vi "ziExample-PWA_SignalInput.vi"() -> ()   [LabVIEW 2009]
doc: "Control a Zurich instrument device via the LabOne Labview API. \nRequirements: Zurich Instruments UHFLI \nThis example retrives Periodic Waveform Analyzer (PWA) data from an UHFLI instrument.\n\n© Zurich Instruments AG, www.zhinst.com\\"
uses:
  <instrlib>/Zurich Instruments LabOne/Public/Data/ziTypePWAWave.ctl
  <instrlib>/Zurich Instruments LabOne/Public/Configure/ziGetValueString.vi
  <instrlib>/Zurich Instruments LabOne/Public/Configure/ziSetValueDoubleArray.vi
  <vilib>/Analysis/2dsp.llb/Real FFT.vi
  <instrlib>/Zurich Instruments LabOne/Public/Data/ziGetEventPWAWave.vi
  <instrlib>/Zurich Instruments LabOne/Zurich Instruments LabOne.lvlib
  <vilib>/Analysis/NI_AALPro.lvlib
  <vilib>/Analysis/NI_AALBase.lvlib
panel:
  out "Error Out":errorcluster
  out "Selected Device":string
  in  "Address":string="DEV"
  in  "Bins":i32=512
  in  "stop":bool
  out "PWAWave":T1={"Timestamp (ticks)"=2149, "SampleCount"=0, "InputSelect"=0, "OscSelect"=0, "Harmonic"=0, "BinCount"=0, "Frequency (Hz)"=0.0, "PWAType"=0, "Mode"=0, "Overflow"=0, "Commensurable"=0, "BinPhase"=[], "X"=[], "Y"=[], "countBin"=[]} {"Frequency (Hz)" format="%#_6p"}
  out "FFT / Harmonics":dbl[](graph)
  out "Waveform":cluster{dbl[], dbl[]}(graph)
  out "Counts per Bin":cluster{dbl[], u32[]}(graph)
  # "ziExample-PWA.vi\nRequirements: UHFLI + BOX\nOptional: MF\nsee block diagram for VI description"
  # "Tested Devices:\n- UHFLI"
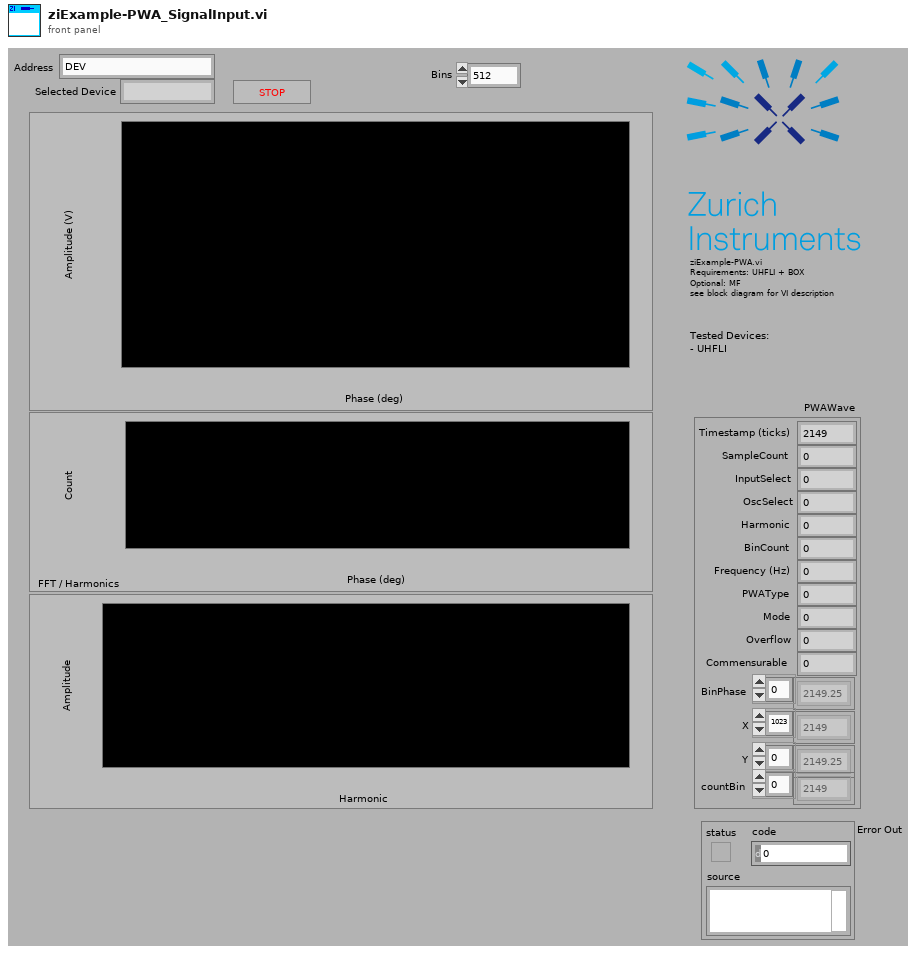
[diagram p1: front panel]
types:
  T1 = typedef "Zurich Instruments LabOne.lvlib/ziTypePWAWave.ctl" = cluster{"Timestamp (ticks)":u64, "SampleCount":u64, "InputSelect":i32, "OscSelect":i32, "Harmonic":i32, "BinCount":i32, "Frequency (Hz)":dbl, "PWAType":u8, "Mode":u8, "Overflow":u8, "Commensurable":u8, "BinPhase":dbl[], "X":dbl[], "Y":dbl[], "countBin":u32[]}
  T2 = typedef "Zurich Instruments LabOne.lvlib/ziTypeHandle.ctl" = cluster{"handleValid":bool, "Conn":u64, "Path Prefix":string, "Handle":u64, "Connected":bool, "Clockbase(s)":dbl}
  T3 = typedef "Zurich Instruments LabOne.lvlib/ziTypePollType.ctl" = enum16{"NONE", "DOUBLE_DATA", "INTEGER_DATA", "DEMOD_SAMPLE", "SCOPE_WAVE_HF2", "AUXIN_SAMPLE", "DIO_SAMPLE", "BYTE_ARRAY", "PWA_WAVE", "9", "10", "11", "12", "13", "14", "15", "TREE_CHANGE_DEPRI", "17", "ERROR", "19", "20", "21", "22", "23", "24", "25", "26", "27", "28", "29", "30", "31", "DOUBLE_DATA_TS", "INTEGER_DATA_TS", "34", "SCOPE_WAVE", "SCOPE_WAVE_EX", "37", "BYTE_ARRAY_TS", "39", "40", "41", "42", "43", "44", "45", "CNT_DATA", "47", "TREE_CHANGE", "49", "50", "51", "52", "53", "54", "55", "56", "57", "58", "59", "60", "61", "62", "63", "SWEEPER_DATA", "SPECTRUM_DATA", "ADVISOR_DATA", "VECTOR_DATA", "IMP_DATA"}
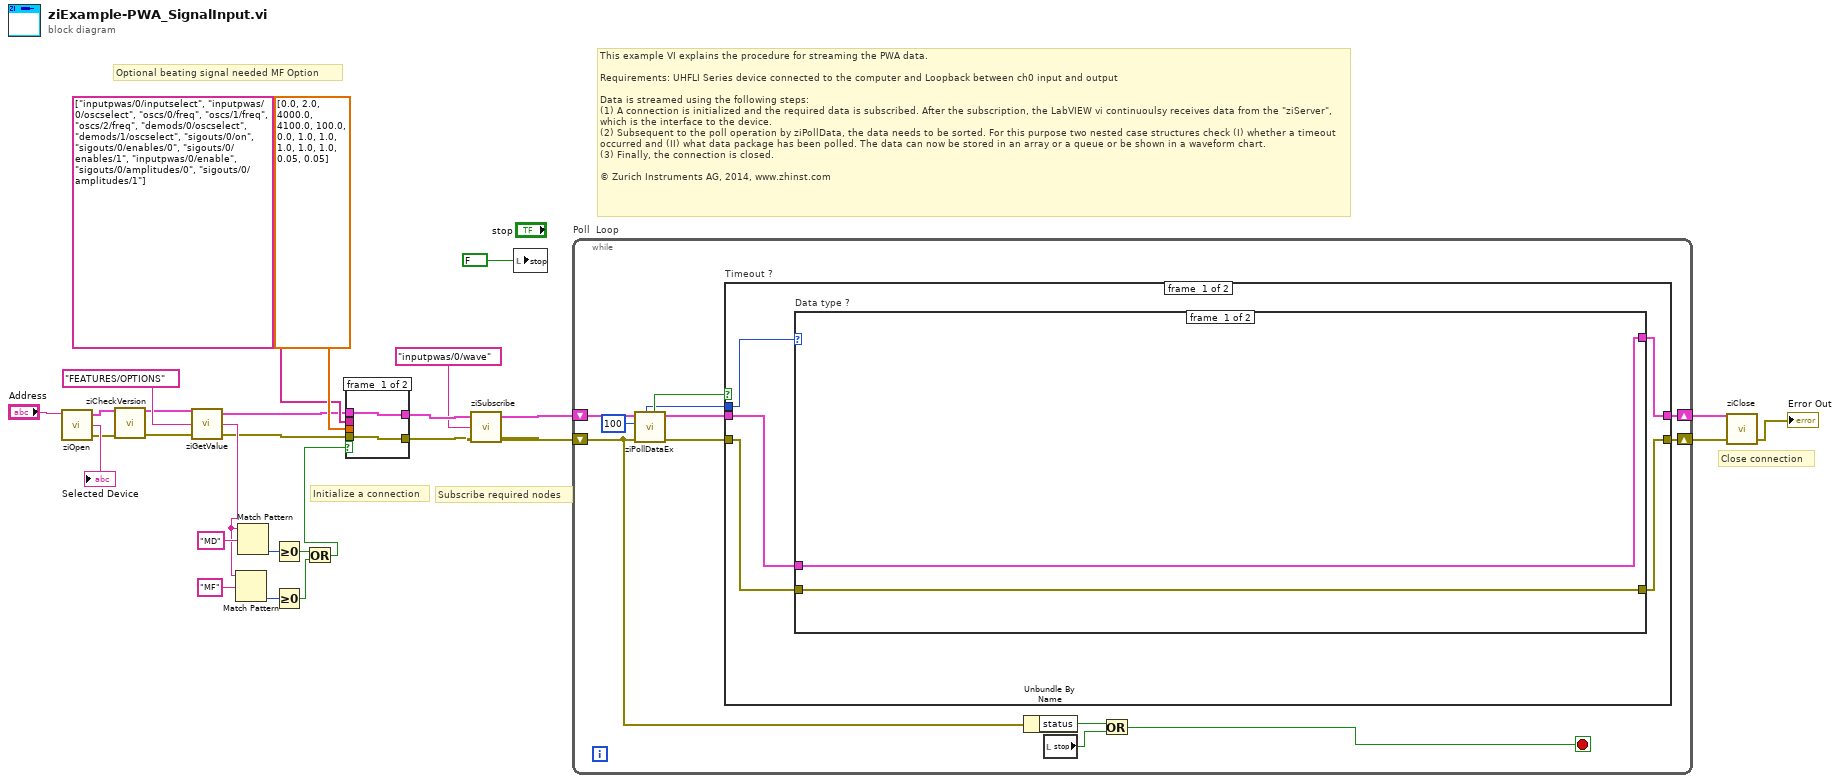
[diagram p0: block diagram]
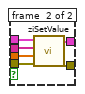
[diagram p2: hidden frame]
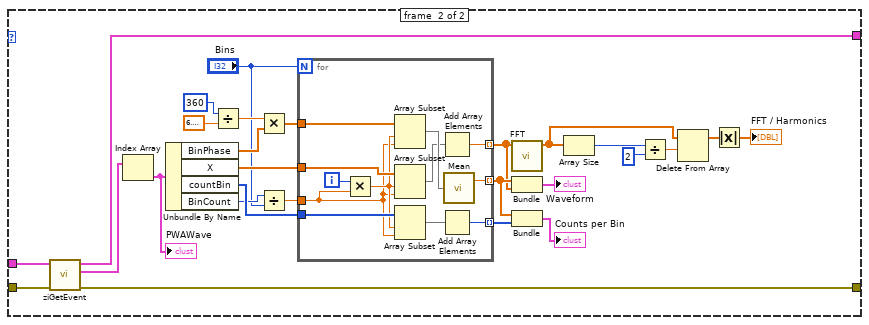
[diagram p3: hidden frame]
diagram:
  # "Optional beating signal needed MF Option"
  # "Close connection"
  # "Initialize a connection"
  # "Subscribe required nodes"
  # "This example VI explains the procedure for streaming the PWA data.\n\nRequirements: UHFLI Series device connected to the computer and Loopback between ch0 input and output\n\nData is streamed using the following steps:\n(1) A connection is initialized and the required data is subscribed. After the subscription, the LabVIEW vi continuoulsy receives data from the \"ziServer\", which is the interface to the device. \n(2) Subsequent to the poll operation by ziPollData, the data needs to be sorted. For this purpose two nested case structures check (I) whether a timeout occurred and (II) what data package has been polled. The data can now be stored in an array or a queue or be shown in a waveform chart. \n(3) Finally, the connection is closed. \n\n© Zurich Instruments AG, 2014, www.zhinst.com"
  n1 = call <instrlib>:"ziOpen.vi"("Address"="Address") -> ("Error Out"=w3:errorcluster, "Selected Device"=→"Selected Device":string, "HandleOut"=w4:T2)  [unwired: 1 in, 2 out]
  n2 = call <instrlib>:"ziCheckVersion.vi"("Handle In"=w4, "Error In"=w3) -> ("Handle Out"=w2:T2, "Error Out"=w1:errorcluster)  [unwired: 11 in, 1 out]
  n3 = call-poly <instrlib>:"ziGetValue.vi"("error in"=w1, "Path"="FEATURES/OPTIONS", "Handle In"=w2) -> ("error out"=w8:errorcluster, "Value"=w13:string, "Handle Out"=w7:T2)
  n4 = Match Pattern(string=w13, regular expression="MF") -> (offset past match=w11:i32)  [unwired: 1 in, 3 out]
  n5 = Match Pattern(string=w13, regular expression="MD") -> (offset past match=w14:i32)  [unwired: 1 in, 3 out]
  n6 = Greater Or Equal To 0?(x=w14) -> (x >= 0?=w10:bool)
  n7 = Greater Or Equal To 0?(x=w11) -> (x >= 0?=w9:bool)
  n8 = Or(x=w10, y=w9) -> (x .or. y?=w6:bool)
  n9 = case shown="True" w6 {
    tunnel: [w30 w36] -> w21
    tunnel: [w29 w35] -> w20
    tunnel: dbl[] [0.0, 2.0, 4000.0, 4100.0, 100.0, 0.0, 1.0, 1.0, 1.0, 1.0, 1.0, 0.05, 0.05] ("abs(x)") -> [_ w34]
    tunnel: string[] ["inputpwas/0/inputselect", "inputpwas/0/oscselect", "oscs/0/freq", "oscs/1/freq", "oscs/2/freq", "demods/0/oscselect", "demods/1/oscselect", "sigouts/0/on", "sigouts/0/enables/0", "sigouts/0/enables/1", "inputpwas/0/enable", "sigouts/0/amplitudes/0", "sigouts/0/amplitudes/1"] -> [_ w33]
    tunnel: w8 -> [w29 w32]
    tunnel: w7 -> [w30 w31]
    frame #0 {
    }
    frame #1 {
      n10 = call-poly <instrlib>:"ziSetValue.vi"("Error In"=w32, "Values"=w34, "Paths"=w33, "Handle In"=w31) -> ("Error Out"=w35:errorcluster, "Handle Out"=w36:T2)  [unwired: 1 in]
    }
  }
  n11 = call <instrlib>:"ziSubscribe.vi"("error in"=w20, "Path ()"="inputpwas/0/wave" ("path"), "Handle In"=w21) -> ("error out"=w24:errorcluster, "Handle Out"=w25:T2)  [unwired: 1 in]
  n12 = local write "stop"(FALSE ("Record")) -> ()
  n13 = while "Poll  Loop" {
    shift-right: [w44] -> w26
    shift-left: w25 -> [w48]
    shift-right: [w42] -> w27
    shift-left: w24 -> [w39]
    stop <- w38 stop-if-true
    n14 = call <instrlib>:"ziPollDataEx.vi"("error in"=w39, "Timeout ms (50)"=100 ("TimeOut ms (50)"), "Handle In"=w48) -> ("error out"=w43:errorcluster, "Handle Out"=w45:T2, "Timed Out"=w46:bool, "ziValueType"=w41:T3)  [unwired: 1 in, 4 out]
    n15 = case "Timeout ?" shown="False" w46 {
      tunnel: w41 -> [w49 _]
      tunnel: w45 -> [w53 w96]
      tunnel: [w52 w96] -> w44
      tunnel: w43 -> [w51 w95]
      tunnel: [w50 w95] -> w42
      frame #0 {
        n16 = case "Data type ?" shown="\"PWA_WAVE\"" w49 {
          tunnel: w53 -> [w55 w82]
          tunnel: [w55 w81] -> w52
          tunnel: w51 -> [w54 w69]
          tunnel: [w54 w68] -> w50
          frame #0 {
          }
          frame #1 {
            n17 = call-poly <instrlib>:"ziGetEvent.vi"("Error In"=w69, "Handle In"=w82) -> ("Error Out"=w68:errorcluster, "PWAWaves Out"=w67:T1[], "Handle Out"=w81:T2)  [unwired: 7 in]
            n18 = Index Array(array=w67) -> (element=w60:T1)  [unwired: 1 in]
            "PWAWave" <- w60
            n19 = Unbundle By Name(w60) -> ("BinPhase"=w58:dbl[], "X"=w59:dbl[], "countBin"=w80:u32[], "BinCount"=w57:i32)
            n20 = Divide(x=360, y=6.283185307179586) -> (x/y=w77:dbl)
            n21 = Multiply(x=w77, y=w58) -> (x*y=w76:dbl[])
            n22 = Divide(x=w57, y="Bins") -> (x/y=w62:dbl)
            n23 = for {
              N: "Bins" -> [_]
              tunnel: w80 -> [w92]
              tunnel: w76 -> [w94]
              tunnel: w59 -> [w88]
              tunnel: w62 -> [w86]
              tunnel: [w84] -> w66 mode=indexing
              tunnel: [w89] -> w65 mode=indexing
              tunnel: [w83] -> w61 mode=indexing
              i -> [w93]
              n24 = Multiply(x=w93, y=w86) -> (x*y=w87:dbl)
              n25 = Array Subset(array=w94, index=w87, length=w86) -> (w90:dbl[])
              n26 = Array Subset(array=w88, index=w87, length=w86) -> (w85:dbl[])
              n27 = Array Subset(array=w92, index=w87, length=w86) -> (w91:u32[])
              n28 = Add Array Elements(numeric array=w85) -> (sum=w83:dbl)
              n29 = Add Array Elements(numeric array=w91) -> (sum=w84:u32)
              n30 = call <vilib>:"Mean.vi"("X"=w90) -> ("mean"=w89:dbl)  [unwired: 1 out]
            }
            n31 = call-poly <vilib>:"FFT.vi"("X"=w61) -> ("FFT {X}"=w73:cdb[])  [unwired: 9 in, 1 out]
            n32 = Bundle(w65, w61) -> (→"Waveform":cluster{dbl[], dbl[]})  [unwired: 1 in]
            n33 = Bundle(w65, w66) -> (→"Counts per Bin":cluster{dbl[], u32[]})  [unwired: 1 in]
            n34 = Array Size(array=w73) -> (size(s)=w72:i32)
            n35 = Divide(x=w72, y=2) -> (x/y=w70:dbl)
            n36 = Delete From Array(array=w73, length=w70) -> (array with subset deleted=w74:cdb[])  [unwired: 1 in, 1 out]
            n37 = Absolute Value(x=w74) -> (abs(x)=→"FFT / Harmonics":dbl[])
          }
        }
      }
      frame #1 {
        # "Timeout, no action."
      }
    }
    n38 = Unbundle By Name(w39) -> ("status"=w40:bool)
    n39 = local read "stop"() -> (w37:bool)
    n40 = Or(x=w40, y=w37) -> (x .or. y?=w38:bool)
  }
  n41 = call <instrlib>:"ziClose.vi"("Error In"=w27, "Handle In"=w26) -> ("Error Out"=→"Error Out":errorcluster)  [unwired: 3 out]
